vi "set_enabled_state.vi"(8 "error in (no error)":errorcluster, 10 "enabled?":bool, 11 "Stimulator090724Scaffold in":refnum<class "Stimulator090724Scaffold.lvclass">) -> (0 "error out":errorcluster, 3 "Stimulator090724Scaffold out":refnum<class "Stimulator090724Scaffold.lvclass">)   [LabVIEW 2010, in "Stimulator090724Scaffold.lvclass"]
uses:
  Stimulator090724Scaffold.lvclass
  Stimulator090724Scaffold.lvclass/Stimulator090724Scaffold.ctl
  Clock/GenericClock/GenericClock/GenericClock.lvclass
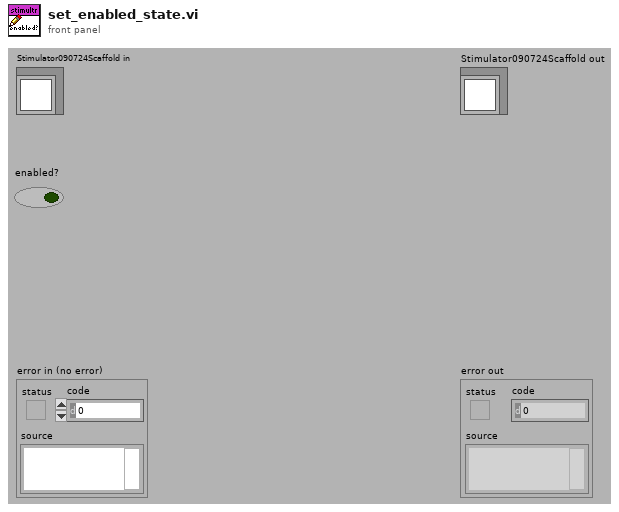
[diagram p1: front panel]
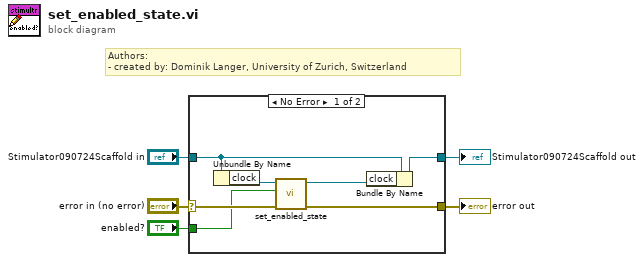
[diagram p0: block diagram]
diagram:
  # "Authors: \n- created by: Dominik Langer, University of Zurich, Switzerland"
  n1 = case shown="No Error" "error in (no error)" {
    selector: "error in (no error)" -> [w10 w13]
    tunnel: "Stimulator090724Scaffold in" -> [w12 w14]
    tunnel: [w8 w13] -> w3
    tunnel: [w11 w14] -> w2
    tunnel: "enabled?" -> [w6 _]
    frame No Error {
      n2 = Unbundle By Name(w12) -> ("clock"=w9:refnum<class "GenericClock.lvclass">)
      n3 = call-dynamic "set_enabled_state.vi"("error in (no error)"=w10, "enabled?"=w6, "GenericClock in"=w9) -> ("error out"=w8:errorcluster, "GenericClock out"=w7:refnum<class "GenericClock.lvclass">)  [unwired: 7 in]
      n4 = Bundle By Name(cluster=w12, "clock"=w7) -> (w11:refnum<class "Stimulator090724Scaffold.lvclass">)
    }
    frame Error {
    }
  }
  "error out" <- w3
  "Stimulator090724Scaffold out" <- w2
